vi "raw data hlr torque.vi"() -> ()   [LabVIEW 2018]
uses:
  <vilib>/FPGAPlugInAG/cRIO-9082/niLvFpga_Open_cRIO-9082.vi
  <vilib>/rvi/interface/common/dynamic/niFpgaDynamicAddResources.vi
  <vilib>/FPGAPlugInAG/Dynamic/niLvFpga_Reset_Dynamic.vi
  <vilib>/FPGAPlugInAG/Dynamic/niLvFpga_Run_Dynamic.vi
  <vilib>/Utility/error.llb/Error Cluster From Error Code.vi
  <vilib>/rvi/errors/niLvFpgaAdjustHostInterfaceError.vi
  <vilib>/FPGAPlugInAG/Dynamic/niLvFpga_Abort_Dynamic.vi
  <vilib>/FPGAPlugInAG/Dynamic/niLvFpga_Close_Dynamic.vi
  <vilib>/rvi/interface/nirviOpenFPGA/nirviOpenFPGA.xnode
  FPGA Bitfiles/new fpga 9082.lvbitx
  <vilib>/rvi/interface/nirviMethod/nirviMethod.xnode
  <vilib>/rvi/interface/nirviReadWriteControl/nirviReadWriteControl.xnode
  <vilib>/rvi/interface/nirviCloseFPGA/nirviCloseFPGA.xnode
  NiFpgaLv.dll
  <vilib>/rvi/interface/Simulation/niFpgaSimulationCallBeginRW.vi
panel:
  in  "stop":bool
  in  "Array":string[](array[string])=["time", "l", "r", "H mode"]
  in  "Headers":string[](array[string])
  in  "error in (no error)":errorcluster
  out "error out":errorcluster
  in  "File Tag":string="actual RAW "
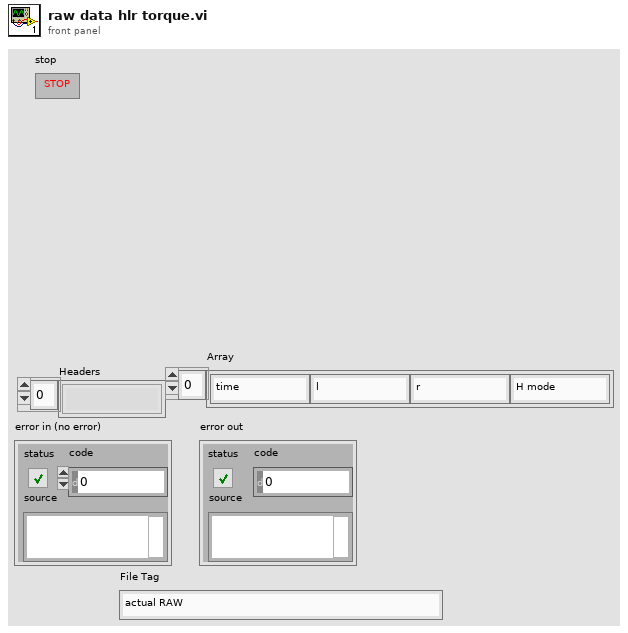
[diagram p1: front panel]
types:
  T1 = enum16{"open", "replace", "create", "open or create", "replace or create", "replace or create with confirmation"}
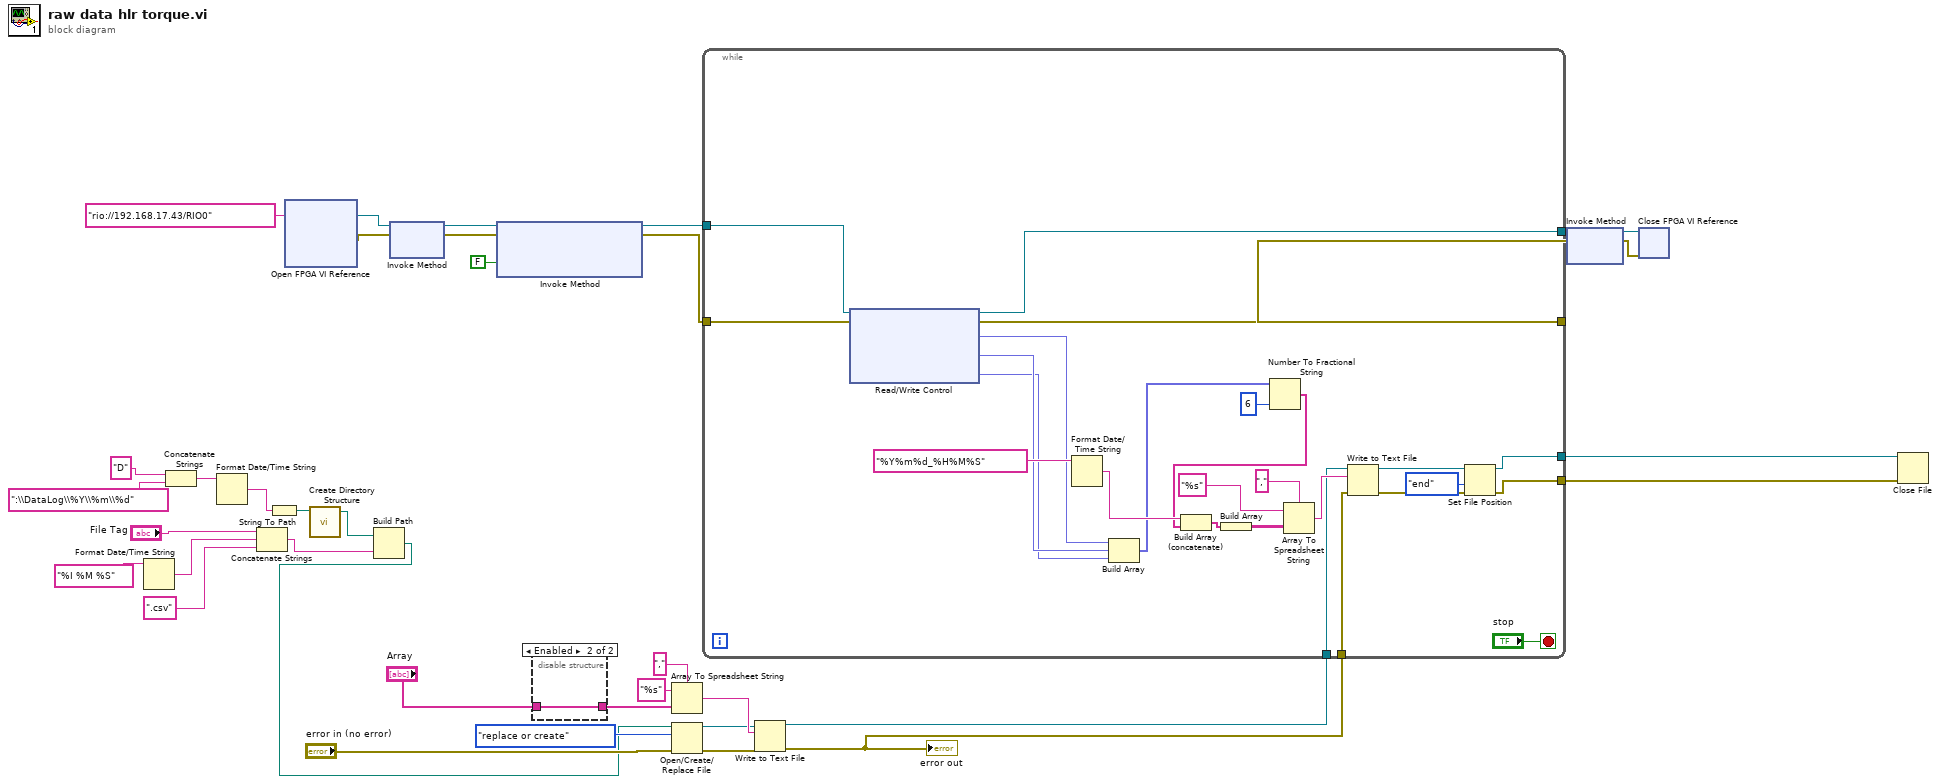
[diagram p0: block diagram]
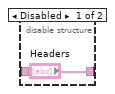
[diagram p2: hidden frame]
diagram:
  n1 = Format Date/Time String(time format string (%c)="%I %M %S") -> (date/time string=w15:string)  [unwired: 2 in]
  n2 = Concatenate Strings("D", ":\\DataLog\\%Y\\%m\\%d") -> (w23:string)
  n3 = Format Date/Time String(time format string (%c)=w23) -> (date/time string=w22:string)  [unwired: 2 in]
  n4 = Concatenate Strings("File Tag", w15, ".csv" ("string")) -> (w20:string)
  n5 = String To Path(string=w22) -> (path=w19:path)
  n6 = xnode "Open FPGA VI Reference"("resource name"=tag "rio://192.168.17.43/RIO0") -> ("FPGA VI Reference Out"=w37:refnum<k20>, "error out"=w36:errorcluster)  [unwired: 1 in]
  n7 = call "Create Directory Structure.vi"("Dir Path In"=w19) -> ("Dir Path Out"=w18:path)  [unwired: 3 in, 1 out]
  n8 = Build Path(base path=w18, name or relative path=w20) -> (appended path=w5:path)
  n9 = xnode "Invoke Method"("FPGA VI Reference In"=w37, "error in"=w36) -> ("FPGA VI Reference Out"=w35:refnum<k20>, "error out"=w34:errorcluster)
  n10 = xnode "Invoke Method"("FPGA VI Reference In"=w35, "error in"=w34, "Wait Until Done (F)"=FALSE) -> ("FPGA VI Reference Out"=w29:refnum<k20>, "error out"=w28:errorcluster)
  n11 = disable-structure shown="Enabled" {
    disable-tunnel: ["Headers" w39] -> w10
    disable-tunnel: "Array" -> [_ w39]
    frame Disabled {
    }
    frame Enabled {
    }
  }
  n12 = Array To Spreadsheet String(delimiter (Tab)=",", array=w10, 3:"%s" ("format string")) -> (spreadsheet string=w11:string)
  n13 = Open/Create/Replace File(file path (use dialog)=w5, error in="error in (no error)", operation (0:open)=T1."replace or create") -> (refnum out=w9:refnum<file>, error out=w7:errorcluster)  [unwired: 3 in, 1 out]
  n14 = Write to Text File(file (use dialog)=w9, text=w11, error in=w7) -> (refnum out=w4:refnum<file>, error out=w3:errorcluster)  [unwired: 1 in, 1 out]
  "error out" <- w3
  n15 = while {
    tunnel: w29 -> [w64]
    tunnel: w28 -> [w63]
    tunnel: [w62] -> w27
    tunnel: [w61] -> w26
    tunnel: w4 -> [w44]
    tunnel: w3 -> [w43]
    tunnel: [w42] -> w2
    tunnel: [w41] -> w1
    stop <- "stop" stop-if-true
    n16 = xnode "Read/Write Control"("FPGA VI Reference In"=w64, "error in"=w63) -> ("FPGA VI Reference Out"=w62:refnum<k20>, "error out"=w61:errorcluster, "Mod8/Torque  L"=w50:fxp<+/-,24,5>, "Mod8/Torque  R"=w49:fxp<+/-,24,5>, "Mod8/Torque  H"=w48:fxp<+/-,24,5>)
    n17 = Format Date/Time String(time format string (%c)="%Y%m%d_%H%M%S") -> (date/time string=w59:string)  [unwired: 2 in]
    n18 = Build Array(w50, w49, w48) -> (w46:fxp<+/-,24,5>[])
    n19 = Number To Fractional String(number=w46, precision (6)=i16 6) -> (F-format string=w45:string[])  [unwired: 2 in]
    n20 = Build Array (concatenate)(w59, w45) -> (w52:string[])
    n21 = Build Array(w52) -> (w51:string[][])
    n22 = Array To Spreadsheet String(delimiter (Tab)=",", array=w51, 3:"%s" ("format string")) -> (spreadsheet string=w53:string)
    n23 = Write to Text File(file (use dialog)=w44, text=w53, error in=w43) -> (refnum out=w58:refnum<file>, error out=w57:errorcluster)  [unwired: 1 in, 1 out]
    n24 = Set File Position(refnum=w58, from (0:start)=enum16{"start", "end", "current"}."end", error in=w57) -> (refnum out=w42:refnum<file>, error out=w41:errorcluster)  [unwired: 1 in]
  }
  n25 = xnode "Invoke Method"("FPGA VI Reference In"=w27, "error in"=w26) -> ("FPGA VI Reference Out"=w31:refnum<k20>, "error out"=w30:errorcluster)
  n26 = xnode "Close FPGA VI Reference"("FPGA VI Reference In"=w31, "error in"=w30) -> ()  [unwired: 1 out]
  n27 = Close File(refnum=w2, error in=w1) -> ()  [unwired: 2 out]
